vi "FTW-DevUtil-CreateNewActor.vi"() -> ()   [LabVIEW 2012]
panel:
  out "error out":errorcluster
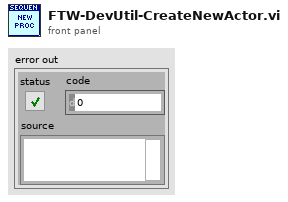
[diagram p1: front panel]
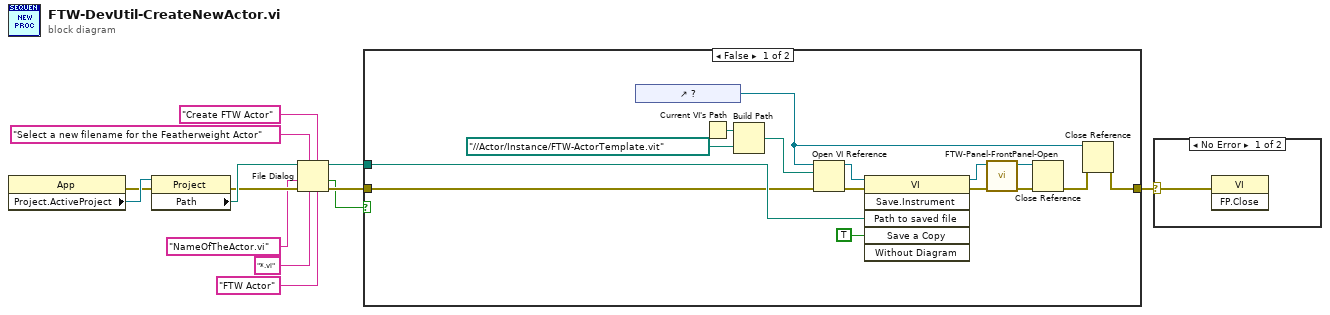
[diagram p0: block diagram]
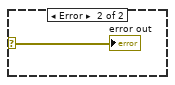
[diagram p2: hidden frame]
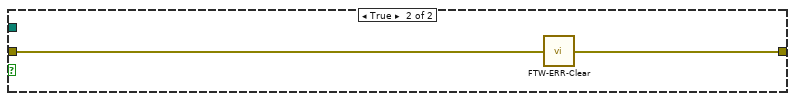
[diagram p3: hidden frame]
diagram:
  n1 = property class="App"() -> (error out=w7:errorcluster, "Project.ActiveProject"=w10:refnum<vi>)  [unwired: 2 in, 1 out]
  n2 = property class="Project"(reference=w10, error in=w7) -> (error out=w8:errorcluster, "Path"=w9:path)  [unwired: 1 out]
  n3 = File Dialog(4:"FTW Actor" ("pattern label"), 5:"Create FTW Actor" ("button label"), 6:"*.vi" ("pattern (all files)"), 7:"Select a new filename for the Featherweight Actor" ("prompt"), 8:w8, 9:"NameOfTheActor.vi" ("default name"), 11:w9) -> (0:w13:errorcluster, 1:w12:bool, 3:w11:path)  [unwired: 1 out]
  n4 = case shown="False" w12 {
    tunnel: [w16 w29] -> w1
    tunnel: w13 -> [w15 w30]
    tunnel: w11 -> [w27 _]
    frame False {
      n5 = control-ref of="?"() -> (w14:refnum<vi>)
      n6 = Current VI's Path() -> (path=w24:path)
      n7 = Build Path(base path=w24, name or relative path=path "../../Actor/Instance/FTW-ActorTemplate.vit" ("vi path")) -> (appended path=w23:path)
      n8 = Open VI Reference(application reference (local)=w14, vi path=w23, error in (no error)=w15) -> (vi reference=w25:refnum<vi>, error out=w26:errorcluster)  [unwired: 3 in]
      n9 = invoke class="VI" method="Save.Instrument"(reference=w25, error in=w26, "Path to saved file"=w27, "Save a Copy"=TRUE) -> (reference out=w18:refnum<vi>, error out=w19:errorcluster)  [unwired: 2 in, 4 out]
      n10 = call "FTW-Panel-FrontPanel-Open.vi"("error in"=w19, "VI Ref"=w18) -> ("error out"=w20:errorcluster, "VI Ref out"=w21:refnum<vi>)  [unwired: 8 in]
      n11 = Close Reference(reference=w21, error in (no error)=w20) -> (error out=w17:errorcluster)
      n12 = Close Reference(reference=w14, error in (no error)=w17) -> (error out=w16:errorcluster)
    }
    frame True {
      n13 = call "FTW-ERR-Clear.vi"("error to snuff"=w30) -> ("no error"=w29:errorcluster)
    }
  }
  n14 = case shown="No Error" w1 {
    selector: w1 -> [w31 w32]
    frame No Error {
      n15 = invoke class="VI" method="FP.Close"(error in=w31) -> ()  [unwired: 2 in, 3 out]
    }
    frame Error {
      "error out" <- w32
    }
  }
